vi "Stepper Set Parameters.vi"(1 "Acceleration Rev/Sec^2":dbl=-1.0 min=-1.0 max=999.0 step=0.01 format="%.2f", 2 "Velocity Rev/Sec":dbl=-1.0 min=0.01 max=50.0 step=0.01 format="%.2f", 3 "error in (no error)":errorcluster, 4 "Encoder":bool, 5 "Motor Number":u32=1 min=1 max=255 step=1, 6 "Instrument Address":refnum<visa-resource-name>) -> (0 "error out":errorcluster)   [LabVIEW 2020]
uses:
  Parker Stepper Global.vi
panel:
  # "Encoder gives lower resolution\n0.36°, but maintains registration when shaft is turned without computer control.  Motor resolution is 0.09° but position is not maintained."
  # "Motor"
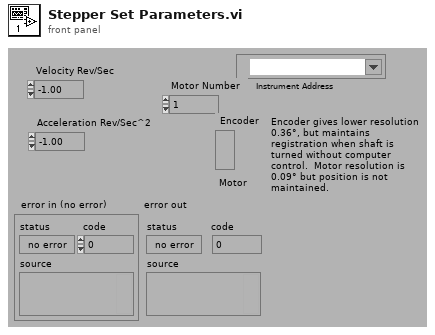
[diagram p1: front panel]
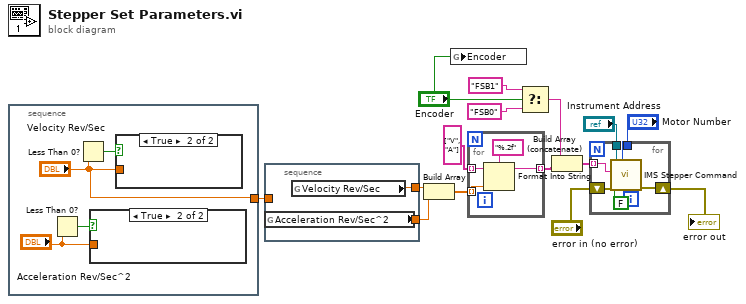
[diagram p0: block diagram]
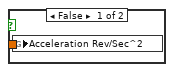
[diagram p2: hidden frame]
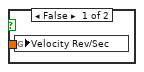
[diagram p3: hidden frame]
diagram:
  n1 = stacked-sequence {
    tunnel: ["Velocity Rev/Sec"] -> w1
    frame #0 {
      n2 = Less Than 0?(x="Acceleration Rev/Sec^2") -> (x < 0?=w18:bool)
      n3 = Less Than 0?(x="Velocity Rev/Sec") -> (x < 0?=w19:bool)
      n4 = case shown="True" w18 {
        tunnel: "Acceleration Rev/Sec^2" -> [w20 _]
        frame False {
          n5 = global write "Parker Stepper Global.vi" "Acceleration Rev/Sec^2"(w20) -> ()
        }
        frame True {
        }
      }
      n6 = case shown="True" w19 {
        tunnel: "Velocity Rev/Sec" -> [w21 _]
        frame False {
          n7 = global write "Parker Stepper Global.vi" "Velocity Rev/Sec"(w21) -> ()
        }
        frame True {
        }
      }
    }
  }
  n8 = stacked-sequence {
    tunnel: [w23] -> w3
    tunnel: [w22] -> w2
    tunnel: w1 -> [_]
    frame #0 {
      n9 = global read "Parker Stepper Global.vi" "Acceleration Rev/Sec^2"() -> (w23:dbl)
      n10 = global read "Parker Stepper Global.vi" "Velocity Rev/Sec"() -> (w22:dbl)
    }
  }
  n11 = Build Array(w2, w3) -> (w11:dbl[])
  n12 = global write "Parker Stepper Global.vi" "Encoder"("Encoder") -> ()
  n13 = for {
    tunnel: w11 -> [w25] mode=indexing
    tunnel: string[] ["V", "A"] -> [w24] mode=indexing
    tunnel: [w27] -> w4 mode=indexing
    n14 = Format Into String(format string="%.2f", initial string=w24, w25) -> (resulting string=w27:string)  [unwired: 1 in, 1 out]
  }
  n15 = Select(t="FSB1", s="Encoder", f="FSB0") -> (s? t:f=w8:string)
  n16 = Build Array (concatenate)(w8, w4) -> (w5:string[])
  n17 = for {
    shift-right: [w32] -> w14
    shift-left: "error in (no error)" -> [w33]
    tunnel: "Instrument Address" -> [w30]
    tunnel: "Motor Number" -> [w29]
    tunnel: w5 -> [w28] mode=indexing
    n18 = call "IMS Stepper Command.vi"("Motor Number"=w29, "error in (no error)"=w33, "Mode"=FALSE, "Command"=w28, "Instrument Address"=w30) -> ("error out"=w32:errorcluster)  [unwired: 1 in, 3 out]
  }
  "error out" <- w14
